vi "Robot Global Data.vi"() -> ()   [LabVIEW 2016]
doc: "This global VI can contain as many global variables as you need. Place a control on the panel, give it a good name. To read or write to it from a VI, drag the icon to the diagram of that VI. You can also drag from the project. Click on the node to change which global you access. You shouldn't have multiple locations writing to a global or it will cause a race-condition."
uses:
  <vilib>/Rock Robotics/WPI/Camera/WPI_CameraImageSize.ctl
  <vilib>/Rock Robotics/WPI/DriverStation/WPI_DriverStationRobotMode2.ctl
  <vilib>/Rock Robotics/WPI/ThirdParty/Sensors/navX/_TypeDefs/FRIC_navX_DeviceNumbersTypeDef.ctl
  <vilib>/Rock Robotics/WPI/ThirdParty/CanMotor/TalonSRX/WPI_CANTalonSRX_APIFeedbackSelect.ctl
panel:
  in  "Camera  Select":bool
  in  "Swerve Calc Command Array":dbl[](array[numeric])
  in  "Drive To Distance Position Cont":bool
  in  "Drive To Distance PID":bool
  in  "Drive to Distance Steps":T1(ring)
  in  "Drive to Distance Direction":enum16{"Y direction", "X Direction"}(ring)
  in  "Drive to Distance Tolerence":dbl
  in  "Drive to Distance setpoint":dbl
  in  "Drive To Distance Complete":bool
  in  "Drive To Distance Enable":bool
  in  "DeadBand":dbl
  in  "Drive Straight out range":cluster{"output high":dbl, "output low":dbl}={"output high"=0.2, "output low"=-0.2}
  in  "Drive Straight PID Gains Sec":T2={"proportional gain (Kc)"=0.01, "integral time (Ti, min)"=0.0, "derivative time (Td, min)"=0.0005}
  in  "Drive Straight PID Gains Pri":T2={"proportional gain (Kc)"=0.01, "integral time (Ti, min)"=0.0, "derivative time (Td, min)"=0.0005}
  in  "Drive Angle min to switch to secondary PID":dbl=5.0
  in  "Drive Angle PID Gains Sec":T2={"proportional gain (Kc)"=0.01, "integral time (Ti, min)"=0.0, "derivative time (Td, min)"=0.0005}
  in  "Shooter PID":dbl[](array[numeric])
  out "Shooter 2 RPM":dbl
  out "Shooter 1 RPM":dbl
  in  "Shoote2 default Speed":dbl=500.0
  in  "Shooter Speed Adjustment":T3(ring)
  in  "Shooter1 default Speed":dbl=500.0
  in  "Shooter2 Speed":dbl
  in  "Shooter1 Speed":dbl
  in  "Shooter Enabled":bool
  in  "Feeder Reverse":bool
  in  "Feeder Speed":dbl
  in  "Feeder Foward":bool
  in  "Winch Speed Direction":dbl
  in  "Winch Enabled":bool
  in  "Joystick 1 Axis":dbl[](array[numeric])
  in  "Joystick 0 Axis":dbl[](array[numeric])
  out "Joystick 1 buttons":bool[](array[boolean])
  out "Joystick 0 buttons":bool[](array[boolean])
  out "Compressor Error":bool
  in  "Gear Holder Open":bool
  out "Compressor Enabled":bool
  out "Compressor Running":bool
  in  "Disable Shortest Distance angle":bool
  in  "Drive Angle out range":cluster{"output high":dbl, "output low":dbl}={"output high"=0.2, "output low"=-0.2}
  in  "Drive angle Time Delay in ms":u32=1000
  out "Test Led":bool
  in  "Drive Yaw Angle SP":dbl
  in  "Drive To angle Tolerence":dbl
  in  "Drive to Angle":bool
  in  "Drive Gearing Red":dbl=1.47
  in  "DriveWheel Dia":dbl=3.25
  in  "Drive Ratio Output":dbl=1.6
  in  "Drive Angle PID Gains  Pri":T2={"proportional gain (Kc)"=0.01, "integral time (Ti, min)"=0.0, "derivative time (Td, min)"=0.0005}
  out "DriveYawControlRunning":bool
  in  "Drive Yaw Straight SP":dbl
  in  "Drive Striaght":bool
  in  "Drive Reset Encoders":bool
  in  "Drive Feedback Reference":T4=enum."CTR Magnetic Enc (Relative)"
  out "RR Drive Rev":bool
  out "RL Drive Rev":bool
  out "FR Drive Rev":bool
  out "FL Drive Rev":bool
  in  "RR Drive RevSensor":bool
  in  "RL Drive RevSensor":bool
  in  "FR Drive RevSensor":bool=TRUE
  in  "FL Drive RevSensor":bool=TRUE
  in  "Drive Encoder PPR":u32=4096
  in  "Steer Angle Commands":dbl[](array[numeric])
  in  "Set Angle to zero for calibration":bool
  in  "Rotate Y vector":dbl
  in  "Rotate X vector":dbl
  in  "Enum":T5(ring)
  in  "SwerveSensorSetting":T6(ring)
  in  "Robot Width":dbl=21.75
  in  "Robot Length":dbl=23.5
  in  "Analog bits Per degree":dbl=2.841
  in  "Swerve Parameters def":T7(ring)
  in  "Target Angle":dbl(knob) scale=-180.0..180.0
  in  "Current Angle":dbl(knob) scale=-180.0..180.0
  in  "Swerve Sensor settings":dbl[][](array[numeric])=[[6.0, 1021.0, 0.0], [6.0, 1023.0, 0.0], [5.0, 1023.0, 0.0], [6.0, 1021.0, 0.0]]
  out "Swerve parameters":dbl[][](array[numeric])
  out "Drive Parameter":dbl[][](array[numeric])
  in  "Swerve Drive Param":T8(ring)
  in  "Drive Settings":dbl[][](array[numeric])=[[0.0, 0.0, 0.0, 0.0, 0.0, 0.0, 0.0, 1.0, -1.0, 0.0], [1.0, 0.0, 0.0, 0.0, 0.0, 0.0, 0.0, 1.0, -1.0, 0.0], [2.0, 0.0, 0.0, 0.0, 0.0, 0.0, 0.0, 1.0, -1.0, 0.0], [3.0, 0.0, 0.0, 0.0, 0.0, 0.0, 0.0, 1.0, -1.0, 0.0], [4.0, 10.0, 0.01, 0.01, 0.0, 30.0, 0.001, 1.0, -1.0, 0.0], [5.0, 10.0, 0.01, 0.01, 0.0, 30.0, 0.001, 1.0, -1.0, 0.0], [6.0, 10.0, 0.01, 0.01, 0.0, 30.0, 0.001, 1.0, -1.0, 0.0], [7.0, 10.0, 0.01, 0.01, 0.0, 30.0, 0.001, 1.0, -1.0, 0.0], [-1.0, -1.0, -1.0, -1.0, -1.0, -1.0, -1.0, -1.0, 0.0, 0.0]]
  in  "axis 3 Z":dbl
  in  "axis 1 X":dbl
  in  "axis 2 Y":dbl
  in  "Set Steer PID":bool
  in  "Analog Encoder Count":dbl=1024.0
  in  "Timer Angle elapsed":u32
  out "Timer Angle  Running":bool
  in  "Timer Angle Enabled":bool
  in  "NavX Device#":T9
  out "Nav Lin Accel Z":dbl
  out "Nav Lin Accel Y":dbl
  out "Nav Lin Accel X":dbl
  out "Nav Disp Z":dbl
  out "Nav Disp Y":dbl
  out "Nav Disp X":dbl
  out "Nav Vel Z":dbl
  out "Nav Vel Y":dbl
  out "Nav Vel X":dbl
  out "Nav Accel Z":dbl
  out "Nav Accel Y":dbl
  out "Nav Accel X":dbl
  out "Nav Fused Heading":dbl
  out "Nav Heading":dbl
  out "Nav Pitch":dbl
  out "Nav Roll":dbl
  out "Nav Yaw":dbl
  in  "Field Concentric Drive":bool
  in  "Nav Reset Vel":bool
  in  "Nav Reset Disp":bool
  in  "Nav Reset Yaw":bool
  out "Nav Connected":bool
  in  "Robot Mode":T10
  in  "image size":T11=enum."320x240"
  in  "Enable Vision":bool
  # "Navagation"
  # "sensor postion\nzero\nrotations\ncalculated angle reading"
  # "SWERVE Drive Parameter"
  # "0 Sensor min value\n1 Sensor max Value\n2 Sensor Position\n3 Closed Loop Error\n4 Rotations\n5 angle\n6 position"
  # "bits/ degree"
  # "Y axis FL,FR,RL,RR\nx axis \nmin value of the encoder\nMax value of encoder full rotation\noffset for wheel zero in count not angle"
  # "L= 23.5  W=21.75\nwheel 3.25"
  # "SWERVE Drive Parameters\nthrottle  encoder opsition"
  # "Row\n0 FL Drive\n1 FR Drive\n2 RL Drive\n3 RR Drive\n4 FL Swerve\n5 FR Swerve\n6 RL Swerve\n7 RR Swerve"
  # "Column\n0 CAN id\n1P\n2 I\n3D\n4 F\n5 I Zone\n6 Ramp Speed\n7 Foward Speed Limit\n8 Rev Speed Limit\n9 Min Sensor pos\n10 Max Sensor Pos"
  # "drive straight Pri \nlow speed travel\ndrive straight sec\nhigh speed travel"
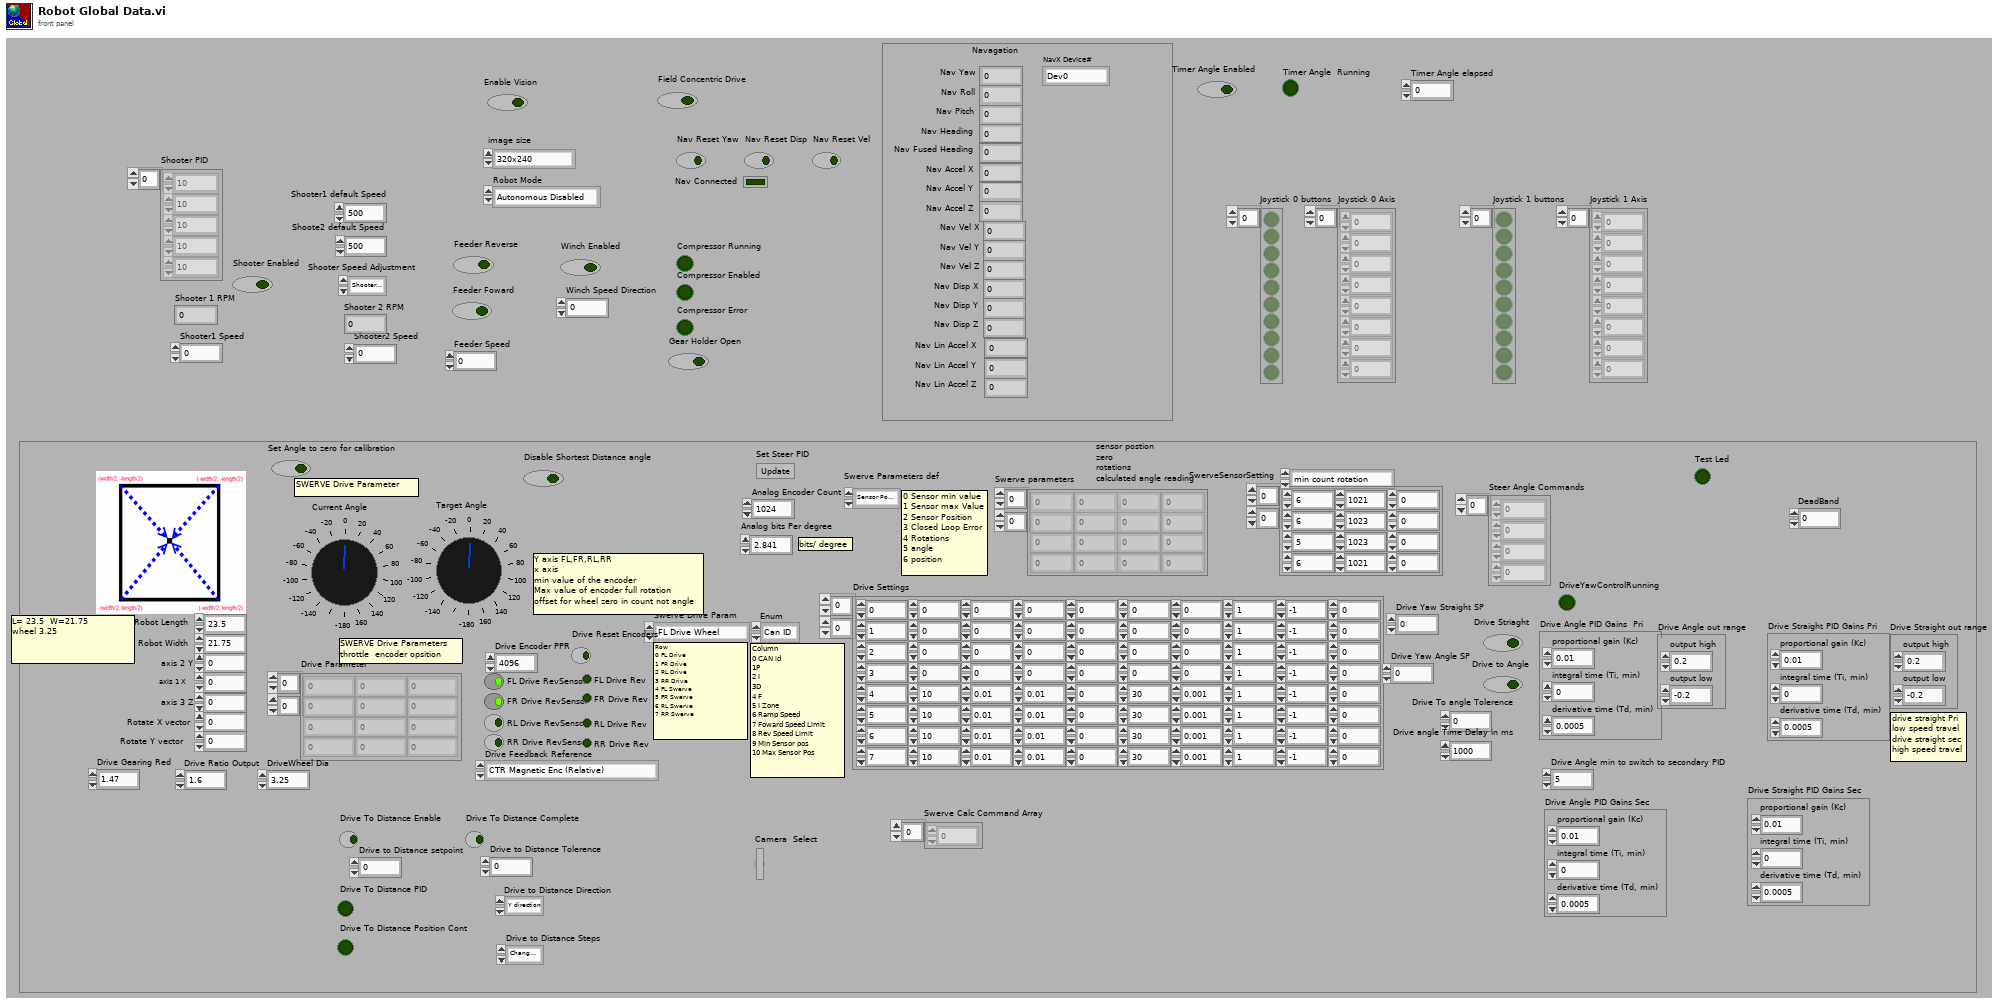
[diagram p1: front panel]
types:
  T1 = enum16{"Change to Position Control", "run the pid loop", "Change the mode back to PWM", ""}
  T2 = cluster{"proportional gain (Kc)":dbl, "integral time (Ti, min)":dbl, "derivative time (Td, min)":dbl}
  T3 = enum16{"Shooter 1 Speed Increase", "Shooter 1 Speed Decrease", "Shooter 2 Speed Increase", "Shooter 2 Speed Decrease", "Nothing Changed", "Set Zero"}
  T4 = typedef "WPI_CANTalonSRX_APIFeedbackSelect.ctl" = enum16{"Digital Quadrature Encoder", "Analog Potentiometer", "Analog Encoder", "Count on Quad-A (Rising-Edge)", "Count on Quad-A (Falling-Edge)", "CTR Magnetic Enc (Absolute)", "CTR Magnetic Enc (Relative)", "Pulse Width"}
  T5 = enum16{"Can ID", "P", "I", "D", "F", "IZone", "RampSpeed", "Fwd speed Limit", "Rev Speed Limit", "InvertDrive"}
  T6 = enum16{"min count rotation", "max count rotation ", "offset count to zero wheel"}
  T7 = enum16{"Sensor Position", "Sensor Velocity", "Rotations", "Angle"}
  T8 = enum16{"FL Drive Wheel", "FR Drive Wheel", "RL Drive Wheel", "RR Drive Wheel", "FL Steer Wheel", "FR Steer Wheel", "RL Steer Wheel", "RR Steer Wheel"}
  T9 = typedef "FRIC_navX_DeviceNumbersTypeDef.ctl" = enum16{"Dev0", "Dev1", "Dev2", "Dev3"}
  T10 = typedef "WPI_DriverStationRobotMode2.ctl" = enum16{"Autonomous Disabled", "Autonomous Enabled", "Teleop Disabled", "Teleop Enabled", "Disconnected", "Finish", "Test Disabled", "Test Enabled", "Emergency Stopped"}
  T11 = typedef "WPI_CameraImageSize.ctl" = enum16{"640x480", "320x240", "160x120", "Custom"}
diagram:
